vi "Exit.vi"(8 "error in (no error)":errorcluster, 11 "queue":refnum<queue>) -> (0 "error out":errorcluster, 3 "queue out":refnum<queue>)   [LabVIEW 2016, in "System Queue.lvlib"]
uses:
  System Queue.lvlib
  Control_Queue Data.ctl
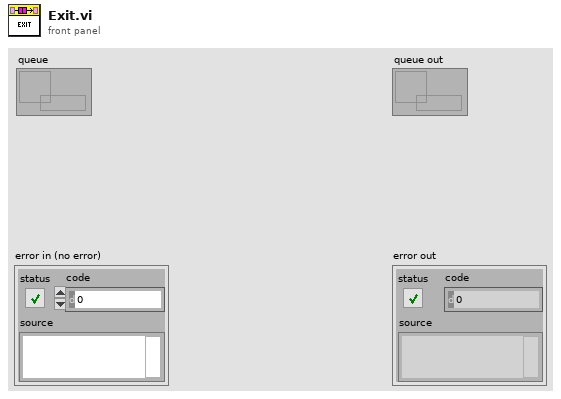
[diagram p1: front panel]
types:
  T1 = typedef "System Queue.lvlib/Control_Queue Data.ctl" = cluster{"Command":string, "Data":variant}
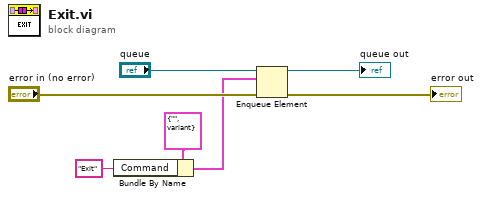
[diagram p0: block diagram]
diagram:
  n1 = Bundle By Name(cluster=T1 {"Command"="", "Data"=variant} ("Queue Data"), "Command"="Exit") -> (w2:T1)
  n2 = Enqueue Element(queue="queue", element=w2, error in (no error)="error in (no error)") -> (queue out=→"queue out":refnum<queue>, error out=→"error out":errorcluster)  [unwired: 1 in, 1 out]
